vi "PDP Graph.vi"(8 "error in":errorcluster, 10 "Timestamp":dbl) -> (0 "error out":errorcluster, 2 "Current":dbl[](array[numeric]))   [LabVIEW 2015]
panel:
  out "40":T1(graph)
  in  "Clear Sticky Faults":bool
  out "Current Faults":bool[](array[boolean])
  out "20/30":T1(graph)
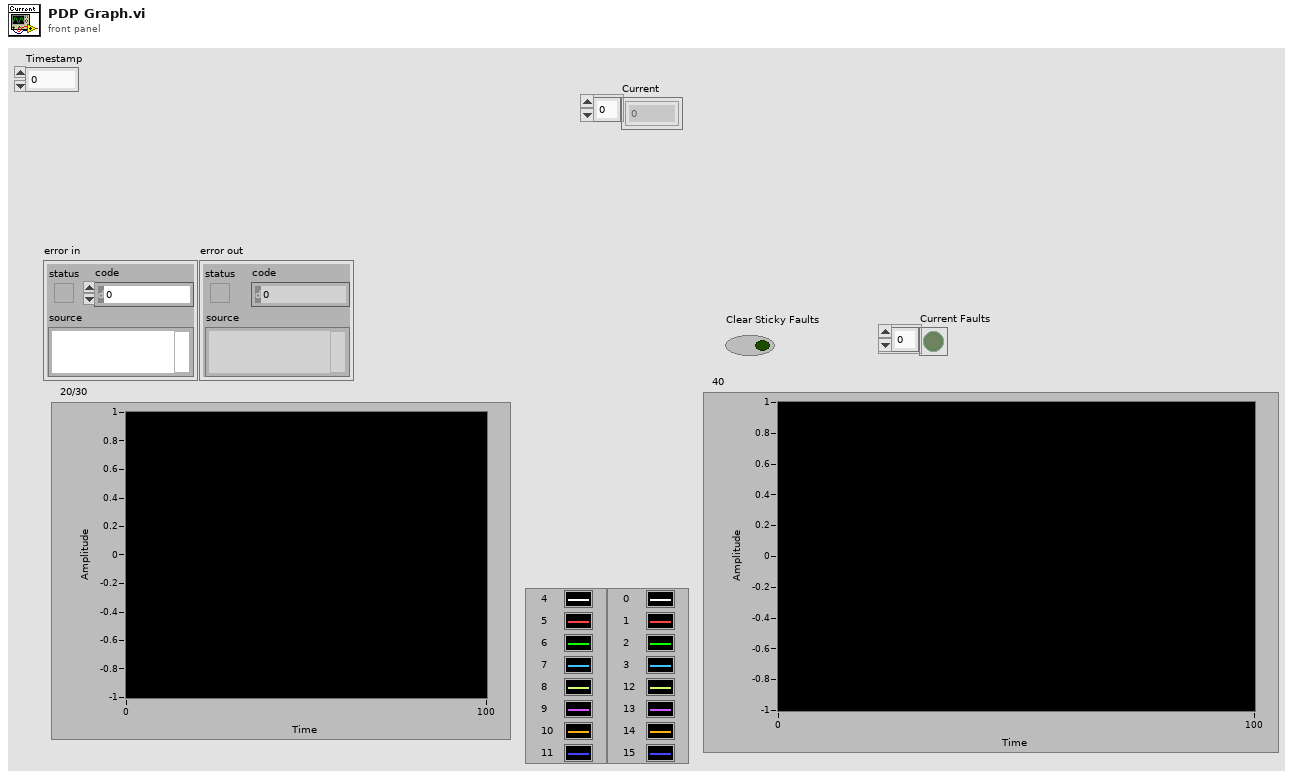
[diagram p1: front panel]
types:
  T1 = cluster{"all currents (A)[4]":dbl, "all currents (A)[5]":dbl, "all currents (A)[6]":dbl, "all currents (A)[7]":dbl, "all currents (A)[8]":dbl, "all currents (A)[9]":dbl, "all currents (A)[10]":dbl, "all currents (A)[11]":dbl}
  T2 = cluster{"all currents (A)[0]":dbl, "all currents (A)[1]":dbl, "all currents (A)[2]":dbl, "all currents (A)[3]":dbl, "all currents (A)[4]":dbl, "all currents (A)[5]":dbl, "all currents (A)[6]":dbl, "all currents (A)[7]":dbl, "all currents (A)[8]":dbl, "all currents (A)[9]":dbl, "all currents (A)[10]":dbl, "all currents (A)[11]":dbl, "all currents (A)[12]":dbl, "all currents (A)[13]":dbl, "all currents (A)[14]":dbl, "all currents (A)[15]":dbl}
  T3 = cluster{"all currents (A)[0]":dbl, "all currents (A)[1]":dbl, "all currents (A)[2]":dbl, "all currents (A)[3]":dbl, "all currents (A)[12]":dbl, "all currents (A)[13]":dbl, "all currents (A)[14]":dbl, "all currents (A)[15]":dbl}
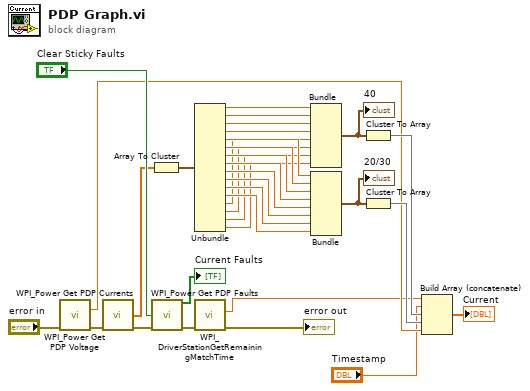
[diagram p0: block diagram]
diagram:
  n1 = call <vilib>:"WPI_Power Get PDP Voltage.vi"("error in"="error in") -> ("voltage (V)"=w3:dbl, "error out"=w4:errorcluster)  [unwired: 13 in]
  n2 = call <vilib>:"WPI_Power Get PDP Currents.vi"("error in"=w4) -> ("all currents (A)"=w30:dbl[], "error out"=w31:errorcluster)  [unwired: 12 in, 1 out]
  n3 = Array To Cluster(array=w30) -> (cluster=w29:T2)
  n4 = call <vilib>:"WPI_Power Get PDP Faults.vi"("Clear Sticky Faults"="Clear Sticky Faults", "error in"=w31) -> ("Current Faults"=→"Current Faults":bool[], "error out"=w8:errorcluster)  [unwired: 9 in, 3 out]
  n5 = Unbundle(w29) -> ("all currents (A)[0]"=w20:dbl, "all currents (A)[1]"=w19:dbl, "all currents (A)[2]"=w18:dbl, "all currents (A)[3]"=w17:dbl, "all currents (A)[4]"=w28:dbl, "all currents (A)[5]"=w27:dbl, "all currents (A)[6]"=w26:dbl, "all currents (A)[7]"=w25:dbl, "all currents (A)[8]"=w24:dbl, "all currents (A)[9]"=w23:dbl, "all currents (A)[10]"=w22:dbl, "all currents (A)[11]"=w21:dbl, "all currents (A)[12]"=w16:dbl, "all currents (A)[13]"=w15:dbl, "all currents (A)[14]"=w14:dbl, "all currents (A)[15]"=w13:dbl)
  n6 = call <vilib>:"WPI_DriverStationGetRemainingMatchTime.vi"("error in (no error)"=w8) -> ("error out"=→"error out":errorcluster, "Match Time(s)"=w1:sgl)  [unwired: 9 in]
  n7 = Bundle("all currents (A)[0]"=w20, "all currents (A)[1]"=w19, "all currents (A)[2]"=w18, "all currents (A)[3]"=w17, "all currents (A)[12]"=w16, "all currents (A)[13]"=w15, "all currents (A)[14]"=w14, "all currents (A)[15]"=w13) -> (w11:T3)  [unwired: 1 in]
  "40" <- w11
  n8 = Bundle("all currents (A)[4]"=w28, "all currents (A)[5]"=w27, "all currents (A)[6]"=w26, "all currents (A)[7]"=w25, "all currents (A)[8]"=w24, "all currents (A)[9]"=w23, "all currents (A)[10]"=w22, "all currents (A)[11]"=w21) -> (w12:T1)  [unwired: 1 in]
  "20/30" <- w12
  n9 = Cluster To Array(cluster=w11) -> (array=w10:dbl[])
  n10 = Cluster To Array(cluster=w12) -> (array=w9:dbl[])
  n11 = Build Array (concatenate)(w1, "Timestamp", w10, w9, w3) -> (→"Current":dbl[])
